vi "Constants.vi"() -> ()   [LabVIEW 2016, in "UDP Custom Device Shared.lvlib"]
doc: "Use this Global VI to access the GUIDs assigned to the page resources of the Custom Device."
uses:
  UDP Custom Device Shared.lvlib
panel:
  in  "Tab Control":enum32{"GUIDS", "Constants", "Properties"}(tab)
  in  "UDP Custom Device":string="fbc40476-d3a5-4e09-a6dd-fa0b6491b895"
  in  "Remote Port":string
  in  "Destination IP Address":string="Destination IP Address"
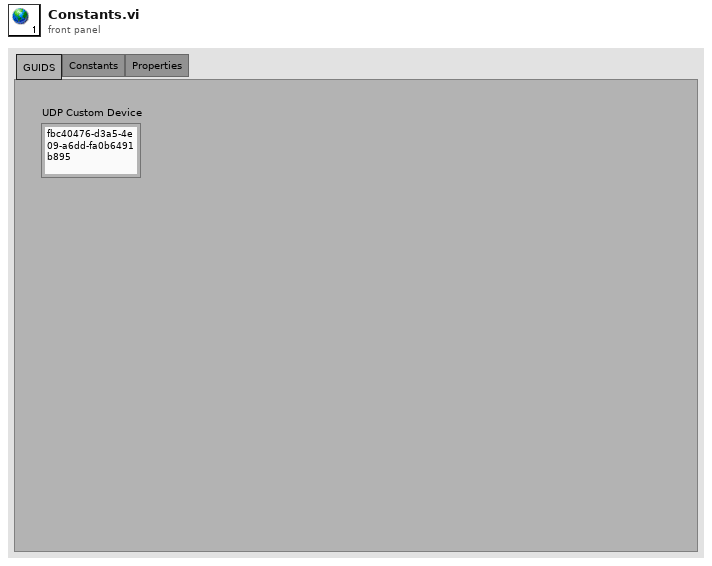
[diagram p1: front panel]
diagram:
